vi "ClusterwitharrayU16.vi"(1 "Cluster In":cluster{"Array In":u16[], "Numeric Input":u16}, 2 "Base":u16) -> (0 "Cluster Out":cluster{"Array Out":u16[], "Numeric Output":u16})   [LabVIEW 2012]
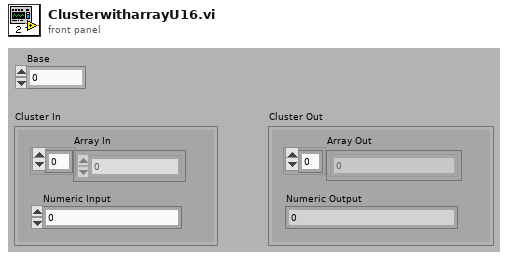
[diagram p1: front panel]
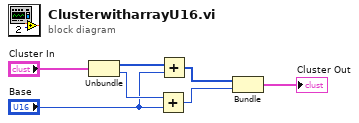
[diagram p0: block diagram]
diagram:
  n1 = Unbundle("Cluster In") -> ("Array In"=w7:u16[], "Numeric Input"=w6:u16)
  n2 = Add(x=w6, y="Base") -> (x+y=w4:u16)
  n3 = Add(x=w7, y="Base") -> (x+y=w5:u16[])
  n4 = Bundle(w5, w4) -> (→"Cluster Out":cluster{u16[], u16})  [unwired: 1 out]
